vi "SingleElementsArray To Data_jkism.vi"(7 "Pototype":variant, 8 "error in (no error)":errorcluster, 11 "DataElementArray":variant[](array[variant])) -> (0 "error out":errorcluster, 3 "Cluster":variant)   [LabVIEW 2017, in "API String Arguments Support.lvlib"]
doc: "This VI converts a DataELementArray to a Cluster."
uses:
  API String Arguments Support.lvlib
  <userlib>/_OpenG.lib/lvdata/lvdata.llb/Type Descriptor Enumeration__ogtk.ctl
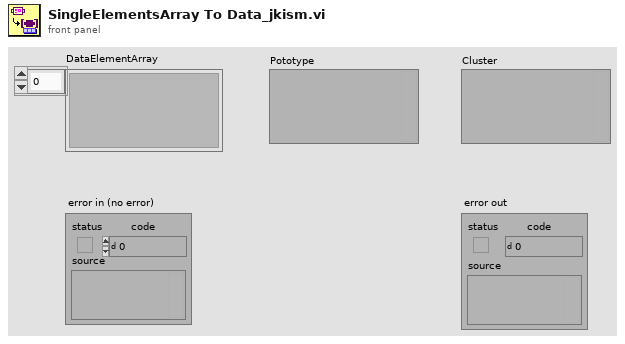
[diagram p1: front panel]
types:
  T1 = typedef "Type Descriptor Enumeration__ogtk.ctl" = enum8{"<Null>", "I8", "I16", "I32", "I64", "U8", "U16", "U32", "U64", "SGL", "DBL", "EXT", "CSG", "CDB", "CXT", "0x0F", "0x10", "0x11", "0x12", "0x13", "0x14", "Enum U8", "Enum U16", "Enum U32", "Enum U64", "SGL PQ", "DBL PQ", "EXT PQ", "CSG PQ", "CDB PQ", "CXT PQ", "0x1F", "0x20", "Boolean", "0x22", "0x23", "0x24", "0x25", "0x26", "0x27", "0x28", "0x29", "0x2A", "0x2B", "0x2C", "0x2D", "0x2E", "0x2F", "String", "0x31", "Path", "Pict", "0x34", "0x35", "0x36", "DAQ", "0x38", "0x39", "0x3A", "0x3B", "0x3C", "0x3D", "0x3E", "0x3F", "Array", "0x41", "0x42", "0x43", "0x44", "0x45", "0x46", "0x47", "0x48", "0x49", "0x4A", "0x4B", "0x4C", "0x4D", "0x4E", "0x4F", "Cluster", "0x51", "0x52", "Variant", "Waveform", "0x55", "0x56", "0x57", "0x58", "0x59", "0x5A", "0x5B", "0x5C", "0x5D", "0x5E", "Fixed Point", "0x60", "0x61", "0x62", "0x63", "0x64", "0x65", "0x66", "0x67", "0x68", "0x69", "0x6A", "0x6B", "0x6C", "0x6D", "0x6E", "0x6F", "Refnum", "0x71", "0x72", "Set Collection", "Map Collection"}
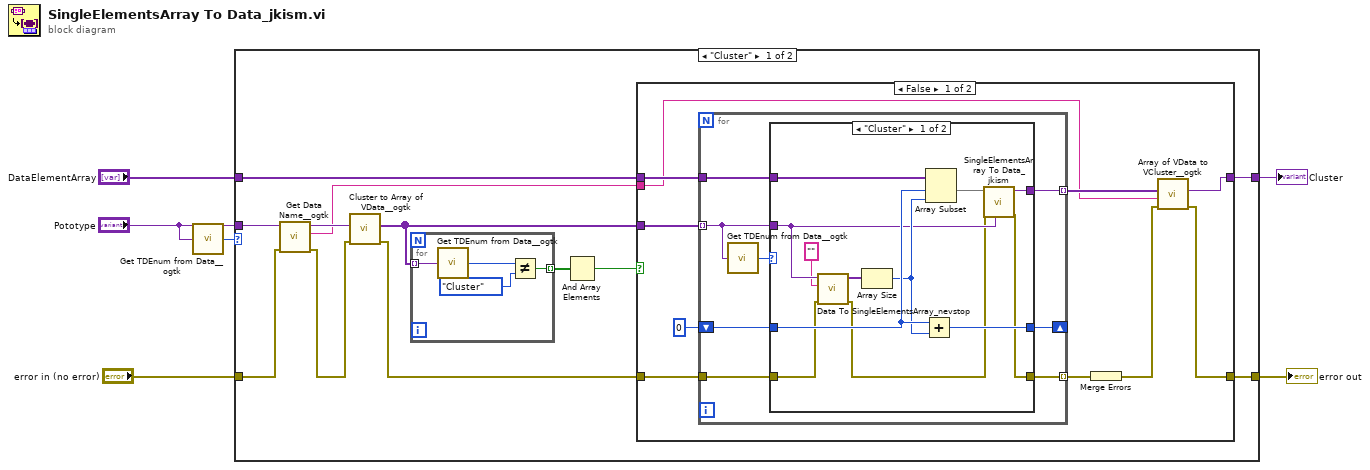
[diagram p0: block diagram]
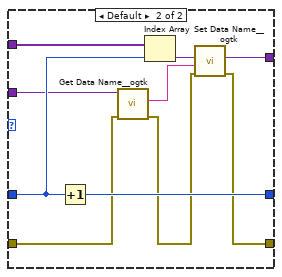
[diagram p2: hidden frame]
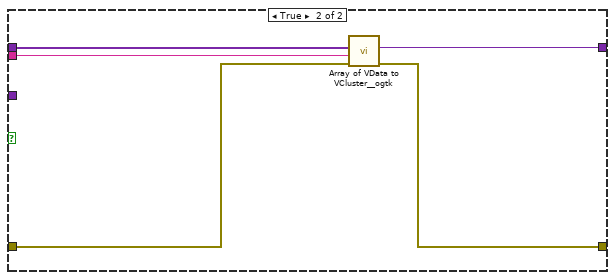
[diagram p3: hidden frame]
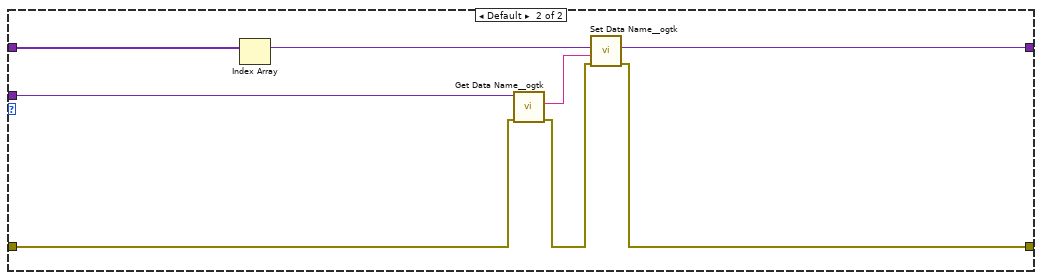
[diagram p4: hidden frame]
diagram:
  n1 = call <userlib>:"Get TDEnum from Data__ogtk.vi"("Data"="Pototype") -> ("Type Descriptor Enumeration"=w6:T1)  [unwired: 4 in]
  n2 = case shown="\"Cluster\"" w6 {
    tunnel: "Pototype" -> [w18 w72]
    tunnel: "DataElementArray" -> [w15 w75]
    tunnel: [w14 w73] -> w3
    tunnel: "error in (no error)" -> [w8 w70]
    tunnel: [w11 w68] -> w1
    frame "Cluster" {
      n3 = call <userlib>:"Get Data Name__ogtk.vi"("error in (no error)"=w8, "Data"=w18) -> ("error out"=w7:errorcluster, "Data Name"=w9:string, "Data dup"=w10:variant)  [unwired: 7 in]
      n4 = call <userlib>:"Cluster to Array of VData__ogtk.vi"("error in (no error)"=w7, "Cluster"=w10) -> ("error out"=w12:errorcluster, "Array of VData"=w13:variant[])  [unwired: 8 in]
      n5 = for {
        tunnel: w13 -> [w67] mode=indexing
        tunnel: [w64] -> w17 mode=indexing
        n6 = call <userlib>:"Get TDEnum from Data__ogtk.vi"("Data"=w67) -> ("Type Descriptor Enumeration"=w66:T1)  [unwired: 4 in]
        n7 = Not Equal?(x=w66, y=Type_Descriptor_Enumeration__ogtk."Cluster") -> (x != y?=w64:bool)
      }
      n8 = And Array Elements(Boolean array=w17) -> (logical AND=w16:bool)
      n9 = case shown="False" w16 {
        tunnel: w15 -> [w24 w63]
        tunnel: [w27 w62] -> w14
        tunnel: w13 -> [w28 _]
        tunnel: w12 -> [w23 w61]
        tunnel: [w19 w60] -> w11
        tunnel: w9 -> [w21 w59]
        frame False {
          n10 = for {
            tunnel: w28 -> [w35] mode=indexing
            tunnel: [w34] -> w26 mode=indexing
            shift-right: [w31] -> _
            shift-left: 0 -> [w32]
            tunnel: w24 -> [w33]
            tunnel: w23 -> [w30]
            tunnel: [w29] -> w22 mode=indexing
            n11 = call <userlib>:"Get TDEnum from Data__ogtk.vi"("Data"=w35) -> ("Type Descriptor Enumeration"=w36:T1)  [unwired: 4 in]
            n12 = case shown="\"Cluster\"" w36 {
              tunnel: w35 -> [w42 w51]
              tunnel: [w48 w52] -> w34
              tunnel: w33 -> [w47 w58]
              tunnel: w32 -> [w46 w57]
              tunnel: [w44 w56] -> w31
              tunnel: w30 -> [w39 w50]
              tunnel: [w37 w49] -> w29
              frame "Cluster" {
                n13 = call <userlib>:"Data To SingleElementsArray_nevstop.vi"("error in (no error)"=w39, "parentUrl"="", "Cluster"=w42) -> ("error out"=w38:errorcluster, "DataElementArray"=w40:variant[])  [unwired: 5 in, 2 out]
                n14 = Array Size(array=w40) -> (size(s)=w45:i32)
                n15 = Add(x=w46, y=w45) -> (x+y=w44:i32)
                n16 = Array Subset(array=w47, index=w46, length=w45) -> (w43:variant[])
                n17 = call "SingleElementsArray To Data_jkism.vi"("Pototype"=w42, "error in (no error)"=w38, "DataElementArray"=w43) -> ("error out"=w37:errorcluster, "Cluster"=w48:variant)  [unwired: 7 in]
              }
              frame Default {
                n18 = Increment(x=w57) -> (x+1=w56:i32)
                n19 = call <userlib>:"Get Data Name__ogtk.vi"("error in (no error)"=w50, "Data"=w51) -> ("error out"=w54:errorcluster, "Data Name"=w55:string)  [unwired: 7 in, 1 out]
                n20 = Index Array(array=w58, index=w57) -> (element=w53:variant)
                n21 = call <userlib>:"Set Data Name__ogtk.vi"("error in (no error)"=w54, "Data Name"=w55, "Data"=w53) -> ("error out"=w49:errorcluster, "Renamed Data"=w52:variant)  [unwired: 7 in]
              }
            }
          }
          n22 = Merge Errors(w22) -> (w20:errorcluster)
          n23 = call <userlib>:"Array of VData to VCluster__ogtk.vi"("error in (no error)"=w20, "Cluster Name"=w21, "Array"=w26) -> ("error out"=w19:errorcluster, "VCluster"=w27:variant)  [unwired: 7 in]
        }
        frame True {
          n24 = call <userlib>:"Array of VData to VCluster__ogtk.vi"("error in (no error)"=w61, "Cluster Name"=w59, "Array"=w63) -> ("error out"=w60:errorcluster, "VCluster"=w62:variant)  [unwired: 7 in]
        }
      }
    }
    frame Default {
      n25 = Index Array(array=w75) -> (element=w74:variant)  [unwired: 1 in]
      n26 = call <userlib>:"Get Data Name__ogtk.vi"("error in (no error)"=w70, "Data"=w72) -> ("error out"=w69:errorcluster, "Data Name"=w71:string)  [unwired: 7 in, 1 out]
      n27 = call <userlib>:"Set Data Name__ogtk.vi"("error in (no error)"=w69, "Data Name"=w71, "Data"=w74) -> ("error out"=w68:errorcluster, "Renamed Data"=w73:variant)  [unwired: 7 in]
    }
  }
  "error out" <- w1
  "Cluster" <- w3
